vi "Zero Gyro.vi"   [LabVIEW 2014]
uses:
  Robot Global Data.vi
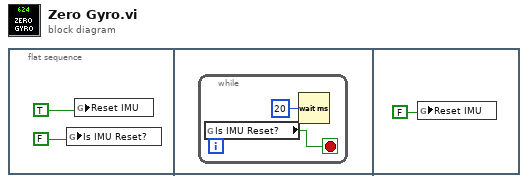
[diagram p0: block diagram]
diagram:
  n1 = flat-sequence {
    frame #0 {
      n2 = global write "Robot Global Data.vi" "Is IMU Reset?"(FALSE ("Reset?")) -> ()
      n3 = global write "Robot Global Data.vi" "Reset IMU"(TRUE ("Reset?")) -> ()
    }
    frame #1 {
      n4 = while {
        stop <- w3 stop-if-true
        n5 = global read "Robot Global Data.vi" "Is IMU Reset?"() -> (w3:bool)
        n6 = Wait (ms)(milliseconds to wait=u32 20) -> ()  [unwired: 1 out]
      }
    }
    frame #2 {
      n7 = global write "Robot Global Data.vi" "Reset IMU"(FALSE ("Reset?")) -> ()
    }
  }
